vi "Test Boolean Omnibus Event.vi"() -> ()   [LabVIEW 2021]
uses:
  Source/Omni-Bus/Omni_Bus.lvclass
  Source/Omni-Bus/Support/Read/Read Boolean.vi
  Source/Event Bus/Event_Bus.lvclass
  Source/Local Bus/Local Bus.lvclass
  <vilib>/Utility/Data Type/Type Definitions/Data Type.ctl
  <vilib>/Utility/Data Type/NI_Data Type.lvlib
  Source/Local Bus/Support/Tag List Type.ctl
  Source/Omni-Bus/Support/Write/Write Boolean.vi
  Source/Event Bus/Support/Event Source/Polled_EventSource/Polled_EventSource.lvclass
  C:/TSA/Omni-Bus/Source/Omni-Bus/Bus Access/Bus_Access.lvclass
  C:/Program Files (x86)/National Instruments/LabVIEW 2021/vi.lib/TSA/Abstract Data Classes/Abs_Types/Type/Abs_Type.lvclass
  C:/TSA/Omni-Bus/Source/Local Bus/Local Bus.lvclass
  C:/TSA/Omni-Bus/Source/Event Bus/Support/Event Source/Event_Source.lvclass
  C:/TSA/Omni-Bus/Source/Event Bus/Support/Event Source/Polled_EventSource/Polled_EventSource.lvclass
  C:/TSA/Omni-Bus/Source/Event Bus/Event_Bus.lvclass
panel:
  in  "Combo Box":string(combo)
  in  "stop 6":bool
  out "Numeric 6":i32
  in  "Boolean 6":bool
  out "Boolean 2":bool
  in  "Boolean":bool
  out "Numeric 2":i32
  out "Numeric":i32
  in  "stop 2":bool
  in  "stop":bool
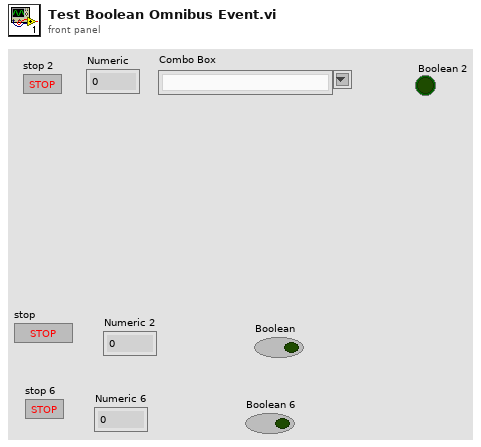
[diagram p1: front panel]
types:
  T1 = typedef "Local Bus.lvclass/Tag List Type.ctl" = cluster{"Tag":string, "Type":T2}
  T2 = typedef "NI_Data Type.lvlib/Data Type.ctl" = enum8{"Invalid Type", "Void", "I8", "I16", "I32", "I64", "U8", "U16", "U32", "U64", "Single Float", "Double Float", "Extended Float", "Single Complex", "Double Complex", "Extended Complex", "Enum U8", "Enum U16", "Enum U32", "Enum U64", "Single Float With Unit", "Double Float With Unit", "Extended Float With Unit", "Single Complex with Unit", "Double Complex with Unit", "Extended Complex with Unit", "Boolean", "String", "Path", "Picture", "Tag", "Array", "Cluster", "Variant", "LV Variant", "Waveform", "Timestamp", "Digital Waveform", "Digital Data", "ExpressData", "Refnum", "External Data", "VI", "Poly VI", "LabVIEW Class Instance", "Fixed Point", "Set Collection", "Map Collection"}
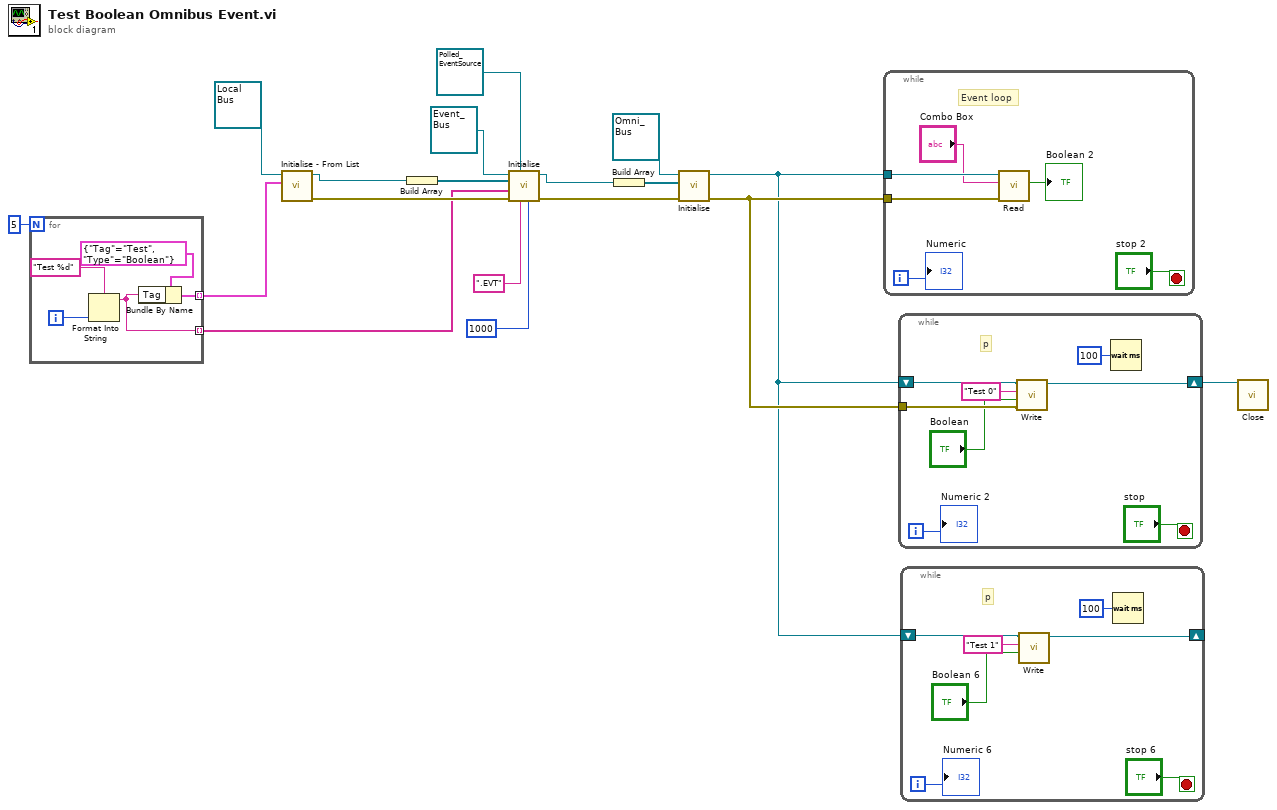
[diagram p0: block diagram]
diagram:
  n1 = for {
    N: 5 -> [_]
    tunnel: [w20] -> w6 mode=indexing
    tunnel: [w19] -> w5 mode=indexing
    i -> [w21]
    n2 = Format Into String(format string="Test %d", w21) -> (resulting string=w19:string)  [unwired: 2 in, 1 out]
    n3 = Bundle By Name(cluster=T1 {"Tag"="Test", "Type"=enum."Boolean"} ("Cluster"), "Tag"=w19) -> (w20:T1)
  }
  n4 = call "Initialise - From List.vi"("Tag List"=w6, "Local Bus in"=refnum<class "Local Bus.lvclass"> refnum) -> ("error out"=w11:errorcluster, "Local Bus out"=w10:refnum<class "Local Bus.lvclass">)  [unwired: 8 in]
  n5 = Build Array(w10) -> (w12:refnum<class "Local Bus.lvclass">[])
  n6 = call "Initialise.vi"("Default Timeout (ms)"=1000, "Tag Root"=".EVT", "Event_Source.lvclass"=refnum<class "Polled_EventSource.lvclass"> refnum ("Polled_EventSource.lvclass"), "error in (no error)"=w11, "Tags to Create Events For"=w5, "Buses"=w12, "Event_Bus in"=refnum<class "Event_Bus.lvclass"> refnum) -> ("error out"=w15:errorcluster, "Event_Bus out"=w14:refnum<class "Event_Bus.lvclass">)  [unwired: 3 in]
  n7 = Build Array(w14) -> (w16:refnum<class "Event_Bus.lvclass">[])
  n8 = call-dynamic "Initialise.vi"("error in (no error)"=w15, "Bus Access"=w16, "Var Bus in"=refnum<class "Omni_Bus.lvclass"> refnum) -> ("error out"=w17:errorcluster, "Var Bus out"=w3:refnum<class "Omni_Bus.lvclass">)  [unwired: 7 in]
  n9 = while {
    tunnel: w3 -> [w29]
    tunnel: w17 -> [w28]
    i -> [w26]
    stop <- "stop 2" stop-if-true
    # "Event loop"
    n10 = call-poly "Read.vi"("error in (no error)"=w28, "Tag"="Combo Box", "Var Bus in"=w29) -> ("Boolean"=→"Boolean 2":bool)  [unwired: 6 in, 2 out]
    "Numeric" <- w26
  }
  n11 = while {
    tunnel: w17 -> [w35]
    shift-right: [w32] -> w8
    shift-left: w3 -> [w36]
    i -> [w34]
    stop <- "stop" stop-if-true
    # "p"
    n12 = call-poly "Write.vi"("error in (no error)"=w35, "Boolean"="Boolean", "Tag"="Test 0", "Omni_Bus in"=w36) -> ("Omni_Bus out"=w32:refnum<class "Omni_Bus.lvclass">)  [unwired: 6 in, 1 out]
    n13 = Wait (ms)(milliseconds to wait=u32 100) -> ()  [unwired: 1 out]
    "Numeric 2" <- w34
  }
  n14 = while {
    shift-right: [w40] -> _
    shift-left: w3 -> [w43]
    i -> [w42]
    stop <- "stop 6" stop-if-true
    # "p"
    n15 = call-poly "Write.vi"("Boolean"="Boolean 6", "Tag"="Test 1", "Omni_Bus in"=w43) -> ("Omni_Bus out"=w40:refnum<class "Omni_Bus.lvclass">)  [unwired: 7 in, 1 out]
    n16 = Wait (ms)(milliseconds to wait=u32 100) -> ()  [unwired: 1 out]
    "Numeric 6" <- w42
  }
  n17 = call-dynamic "Close.vi"("Data in"=w8) -> ()  [unwired: 9 in, 2 out]
